vi "WS_INICIAR.vi"(7 "LabVIEW Web Service Request":refnum<class "Web Request.lvclass">) -> (2 "body":string)   [LabVIEW 2017]
uses:
  <vilib>/wsapi/Web Request.lvclass
  <vilib>/httpClient/LabVIEWHTTPClient.lvlib
panel:
  # "Use the Web Service Request input terminal to call the VIs on the Web Services palette. Do not remove it from the connector pane unless you don't need access to the palette."
  # "Each additional control wired to the connector pane will be available as an input in the URL. To include an indicator in terminal-mode output (the default setting), it must also be wired to the connector pane."
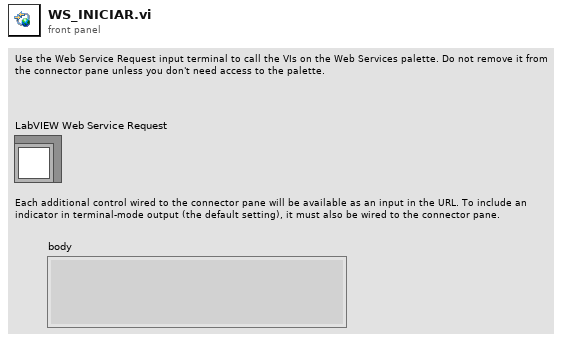
[diagram p1: front panel]
types:
  T1 = typedef "LabVIEWHTTPClient.lvlib/ClientHandle.ctl" = refnum<k1>
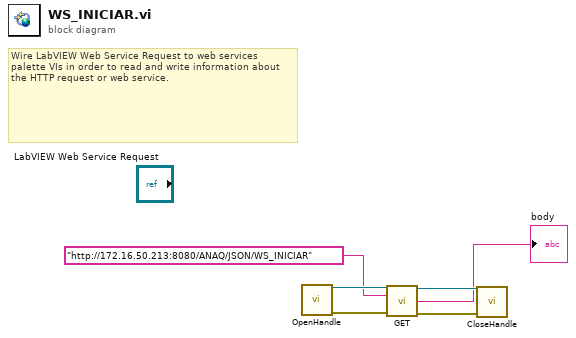
[diagram p0: block diagram]
diagram:
  # "Wire LabVIEW Web Service Request to web services palette VIs in order to read and write information about the HTTP request or web service."
  n1 = call <vilib>:"OpenHandle.vi"() -> ("client handle out"=w6:T1, "error out"=w4:errorcluster)  [unwired: 14 in]
  n2 = call <vilib>:"GET.vi"("client handle"=w6, "url"="http://172.16.50.213:8080/ANAQ/JSON/WS_INICIAR", "error in (no error)"=w4) -> ("client handle out"=w5:T1, "body"=→"body":string, "error out"=w3:errorcluster)  [unwired: 9 in, 1 out]
  n3 = call <vilib>:"CloseHandle.vi"("client handle"=w5, "error in (no error)"=w3) -> ()  [unwired: 13 in, 1 out]
